vi "Add MeasLink Controls.vi"(11 "error in (no error)":errorcluster) -> (15 "error out":errorcluster)   [LabVIEW 2021, in "Migrator.lvlib"]
uses:
  Migrator.lvlib
  Path Functions/Path Functions.lvlib
  Migrator Reusables/Migrator Reusables.lvlib
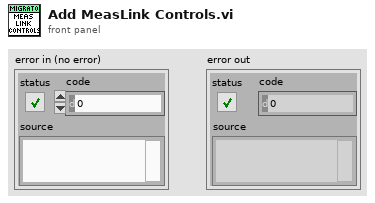
[diagram p1: front panel]
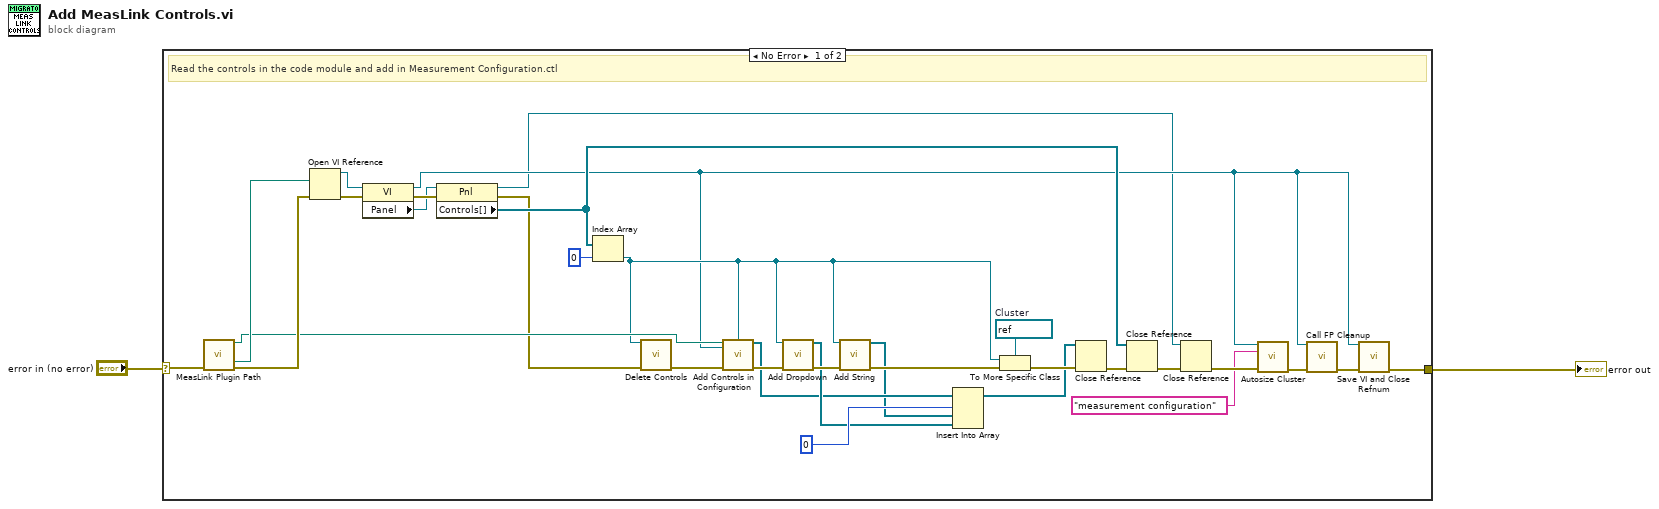
[diagram p0: block diagram]
diagram:
  n1 = case shown="No Error" "error in (no error)" {
    selector: "error in (no error)" -> [w23 w35]
    tunnel: [w29 w35] -> w1
    frame No Error {
      w28 = refnum<vi> refnum  # Cluster
      # "Read the controls in the code module and add in Measurement Configuration.ctl"
      n2 = call "MeasLink Plugin Path.vi"("error in (no error)"=w23) -> ("New Code Module"=w16:path, "Input Controls"=w22:path, "error out"=w24:errorcluster)  [unwired: 2 in, 10 out]
      n3 = Open VI Reference(vi path=w22, error in (no error)=w24) -> (vi reference=w6:refnum<vi>, error out=w30:errorcluster)  [unwired: 4 in]
      n4 = property class="VI"(reference=w6, error in=w30) -> (reference out=w5:refnum<vi>, error out=w34:errorcluster, "Panel"=w4:refnum<vi>)
      n5 = property class="Pnl"(reference=w4, error in=w34) -> (reference out=w3:refnum<vi>, error out=w14:errorcluster, "Controls[]"=w20:refnum<vi>[])
      n6 = Index Array(array=w20, index=0) -> (element=w13:refnum<vi>)
      n7 = call "Delete Controls.vi"("Control in"=w13, "error in (no error)"=w14) -> ("error out"=w15:errorcluster)  [unwired: 13 in]
      n8 = call "Add Controls in Configuration.vi"("New Code Module"=w16, "vi reference"=w5, "Configuration Ctl Refnum"=w13, "error in (no error)"=w15) -> ("Controls Reference"=w9:refnum<vi>[], "error out"=w17:errorcluster)  [unwired: 10 in]
      n9 = call "Add Dropdown.vi"("Control in"=w13, "error in (no error)"=w17) -> ("ComboBox out"=w10:refnum<vi>[], "error out"=w11:errorcluster)  [unwired: 12 in]
      n10 = call "Add String.vi"("Control in"=w13, "error in (no error)"=w11) -> ("ComboBox out"=w7:refnum<vi>[], "error out"=w12:errorcluster)  [unwired: 12 in]
      n11 = Insert Into Array(array=w9, index=0, new element #1=w7, new element #2=w10) -> (w8:refnum<vi>[])
      n12 = To More Specific Class(target class=w28, reference=w13, error in=w12) -> (error out=w26:errorcluster)  [unwired: 1 out]
      n13 = Close Reference(reference=w8, error in (no error)=w26) -> (error out=w19:errorcluster)
      n14 = Close Reference(reference=w20, error in (no error)=w19) -> (error out=w18:errorcluster)
      n15 = Close Reference(reference=w3, error in (no error)=w18) -> (error out=w32:errorcluster)
      n16 = call "Autosize Cluster.vi"("VI Refnum"=w5, "name"="measurement configuration" ("name/order"), "error in (no error)"=w32) -> ("error out"=w21:errorcluster)  [unwired: 12 in]
      n17 = call "Call FP Cleanup.vi"("VI"=w5, "error in (no error)"=w21) -> ("error out"=w25:errorcluster)  [unwired: 13 in]
      n18 = call "Save VI and Close Refnum.vi"("VI Refnum"=w5, "error in"=w25) -> ("error out"=w29:errorcluster)  [unwired: 13 in]
    }
    frame Error {
    }
  }
  "error out" <- w1
